vi "DSF.Engine.Plugin.Tx.Async.vi"(8 "error in (no error)":errorcluster, 11 "Plugin in":refnum<class "DSF.Engine.Plugin.lvclass">) -> (0 "error out":errorcluster, 3 "Plugin out":refnum<class "DSF.Engine.Plugin.lvclass">)   [LabVIEW 2017, in "DSF.Engine.lvlib" / "DSF.Engine.Plugin.lvclass"]
uses:
  DSF.Engine.Plugin.lvclass
  DSF.Engine.Plugin.lvclass/DSF.Engine.Plugin.ctl
  Timing/DSF.Engine.Timing.lvclass/DSF.Engine.Timing.ctl
  Transfer/DSF.Engine.Transfer Group.lvclass/DSF.Engine.Transfer Group.ctl
  Interface/DSF.Engine.Interface.Transceiver.Command.ctl
  Debug/DSF.Engine.Debug Flags.lvclass/DSF.Engine.Debug Flags.ctl
  Debug/DSF.Engine.Debug Flags.FIFO.lvclass/DSF.Engine.Debug Flags.FIFO.ctl
  Transfer/DSF.Engine.Transfer.lvclass/DSF.Engine.Transfer.ctl
  Timing/DSF.Engine.Timing.Is Active Cycle.vi
  Transfer/DSF.Engine.Transfer Group.Return FIFO.Read.vi
  Transfer/DSF.Engine.Transfer Group.Get Transfers.vi
  Transfer/DSF.Engine.Transfer.Get Inline Buffer.vi
  Transfer/DSF.Engine.Transfer.Get Intermediate Buffer.vi
  Timing/DSF.Engine.Timing.Iteration.Increment.vi
  Timing/DSF.Engine.Timing.Get Decimation.vi
  Timing/DSF.Engine.Timing.Get Offset.vi
  Transfer/DSF.Engine.Transfer Group.Get Return FIFO.vi
  Transfer/DSF.Engine.Transfer Group.Get Debug Flags.vi
  Debug/DSF.Engine.Debug Flags.Get FIFO Flags.vi
  Debug/DSF.Engine.Debug Flags.FIFO.Get Infinite Timeouts.vi
  Pointer/DSF.Engine.Pointer.DBL.lvclass
  C:/Git/DSF/DSF Core/Built/PharLap x86/Dependencies/c/Memory Manager.lvlibp/1abvi3w/vi.lib/National Instruments/Memory Manager/Classes/Pointer/Memory.Pointer.lvclass
  Transfer/DSF.Engine.Transfer Group.Errors.vi
  Transfer/DSF.Engine.Transfer Group.Errors.Return Timeout.vi
  Built/Core/Memory Manager.lvlibp/1abvi3w/vi.lib/National Instruments/Memory Manager/Classes/Pointer/Memory.Pointer.Copy All.vi
  Transfer/DSF.Engine.Transfer Group.lvclass
  Timing/DSF.Engine.Timing.lvclass
  Interface/DSF.Engine.Interface.Transceiver.lvclass
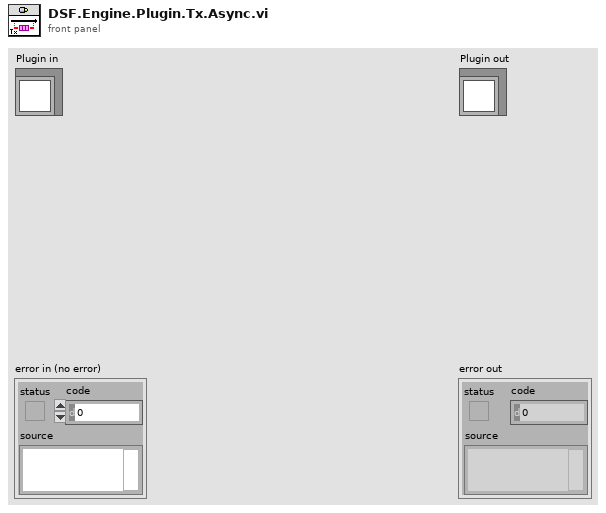
[diagram p1: front panel]
types:
  T1 = typedef "DSF.Engine.lvlib/DSF.Engine.Interface.Transceiver.lvclass/DSF.Engine.Interface.Transceiver.Command.ctl" = enum8{"Set Base Pointer", "Rx", "Tx", "Shutdown"}
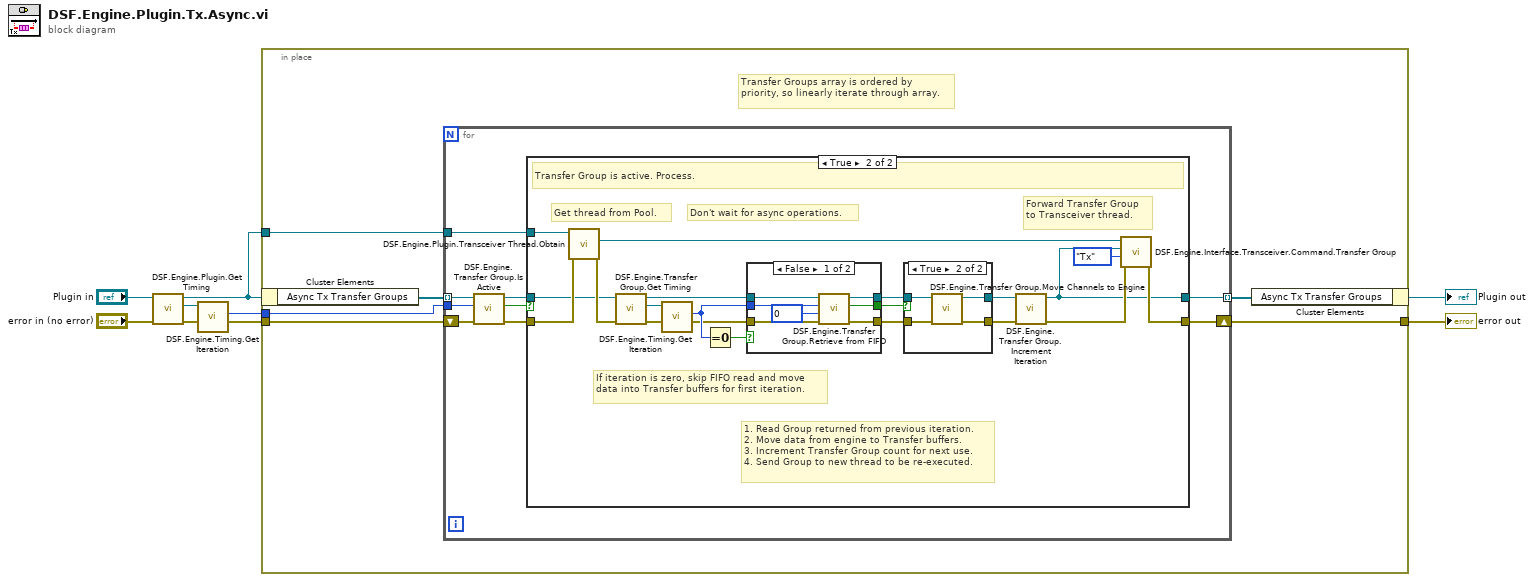
[diagram p0: block diagram]
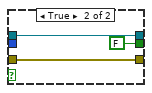
[diagram p3: hidden frame]
diagram:
  n1 = call "DSF.Engine.Plugin.Get Timing.vi"("Plugin in"="Plugin in") -> ("Timing"=w6:refnum<class "DSF.Engine.Timing.lvclass">, "Plugin out"=w7:refnum<class "DSF.Engine.Plugin.lvclass">)  [unwired: 9 in]
  n2 = call "DSF.Engine.Timing.Get Iteration.vi"("Timing in"=w6) -> ("Iteration"=w5:u64)  [unwired: 9 in, 1 out]
  n3 = in-place {
    in-place-border: w7 -> [w13]
    in-place-border: w5 -> [w12]
    in-place-border: "error in (no error)" -> [w11]
    in-place-border: [w10] -> w2
    # "Transfer Groups array is ordered by priority, so linearly iterate through array."
    n4 = in-place-cluster #1(w7) -> ("Async Tx Transfer Groups"=w9:refnum<class "DSF.Engine.Transfer Group.lvclass">[])
    n5 = for {
      tunnel: w9 -> [w21] mode=indexing
      tunnel: w12 -> [w20]
      shift-right: [w14] -> w10
      shift-left: w11 -> [w19]
      tunnel: [w15] -> w8 mode=indexing
      tunnel: w13 -> [w16]
      n6 = call "DSF.Engine.Transfer Group.Is Active.vi"("cycle count"=w20, "Transfer Group in"=w21) -> ("active this cycle?"=w18:bool, "Transfer Group out"=w17:refnum<class "DSF.Engine.Transfer Group.lvclass">)  [unwired: 8 in]
      n7 = case shown="True" w18 {
        tunnel: [w23 w26] -> w14
        tunnel: w19 -> [w23 w30]
        tunnel: w17 -> [w22 w28]
        tunnel: w16 -> [_ w40]
        tunnel: [w22 w25] -> w15
        frame False {
          # "Transfer Group is not active. Skip."
        }
        frame True {
          # "Don't wait for async operations."
          # "If iteration is zero, skip FIFO read and move data into Transfer buffers for first iteration."
          # "Forward Transfer Group to Transceiver thread."
          # "Get thread from Pool."
          # "1. Read Group returned from previous iteration.\n2. Move data from engine to Transfer buffers.\n3. Increment Transfer Group count for next use.\n4. Send Group to new thread to be re-executed."
          # "Transfer Group is active. Process."
          n8 = call "DSF.Engine.Plugin.Transceiver Thread.Obtain.vi"("error in (no error)"=w30, "Plugin in"=w40) -> ("error out"=w29:errorcluster, "Transceiver Thread"=w41:refnum<class "DSF.Engine.Interface.Transceiver.lvclass">)  [unwired: 7 in, 1 out]
          n9 = call "DSF.Engine.Transfer Group.Get Timing.vi"("Transfer Group in"=w28) -> ("Timing"=w38:refnum<class "DSF.Engine.Timing.lvclass">, "Transfer Group out"=w39:refnum<class "DSF.Engine.Transfer Group.lvclass">)  [unwired: 9 in]
          n10 = call "DSF.Engine.Timing.Get Iteration.vi"("Timing in"=w38) -> ("Iteration"=w37:u64)  [unwired: 9 in, 1 out]
          n11 = Equal To 0?(x=w37) -> (x = 0?=w36:bool)
          n12 = case shown="False" w36 {
            tunnel: w29 -> [w48 w50]
            tunnel: [w47 w51] -> w34
            tunnel: [w46 w50] -> w33
            tunnel: w39 -> [w45 w51]
            tunnel: w37 -> [w44 _]
            tunnel: [w43 FALSE ("iteration valid?")] -> w35
            frame False {
              n13 = call "DSF.Engine.Transfer Group.Retrieve from FIFO.vi"("error in (no error)"=w48, "timeout in ms (0)"=0, "expected iteration"=w44, "Transfer Group in"=w45) -> ("error out"=w46:errorcluster, "iteration valid?"=w43:bool, "Transfer Group out"=w47:refnum<class "DSF.Engine.Transfer Group.lvclass">)  [unwired: 5 in]
            }
            frame True {
            }
          }
          n14 = case shown="True" w35 {
            tunnel: w34 -> [w53 w57]
            tunnel: w33 -> [w52 w56]
            tunnel: [w53 w55] -> w32
            tunnel: [w52 w54] -> w31
            frame False {
            }
            frame True {
              n15 = call "DSF.Engine.Transfer Group.Move Channels to Engine.vi"("error in (no error)"=w56, "Transfer Group in"=w57) -> ("error out"=w54:errorcluster, "Transfer Group out"=w55:refnum<class "DSF.Engine.Transfer Group.lvclass">)  [unwired: 8 in]
            }
          }
          n16 = call "DSF.Engine.Transfer Group.Increment Iteration.vi"("error in (no error)"=w31, "Transfer Group in"=w32) -> ("error out"=w27:errorcluster, "Transfer Group out"=w25:refnum<class "DSF.Engine.Transfer Group.lvclass">)  [unwired: 8 in]
          n17 = call "DSF.Engine.Interface.Transceiver.Command.Transfer Group.vi"("error in (no error)"=w27, "Command"=DSF.Engine.Interface.Transceiver.Command."Tx", "Transfer Group"=w25, "Transceiver Interface in"=w41) -> ("error out"=w26:errorcluster)  [unwired: 6 in, 1 out]
        }
      }
    }
    n18 = in-place-cluster #1("Async Tx Transfer Groups"=w8) -> (→"Plugin out":refnum<class "DSF.Engine.Plugin.lvclass">)
  }
  "error out" <- w2
